vi "XNET Write (State Ethernet Sleep).vi"(0 "session in":refnum<k21>, 11 "error in (no error)":errorcluster) -> (4 "session out":refnum<k21>, 15 "error out":errorcluster)   [LabVIEW 2018]
doc: "Writes a request for the local Ethernet interface and its remote link partner to sleep. You can use this XNET Write VI with any input or output session for Ethernet."
uses:
  nixlvapi.dll
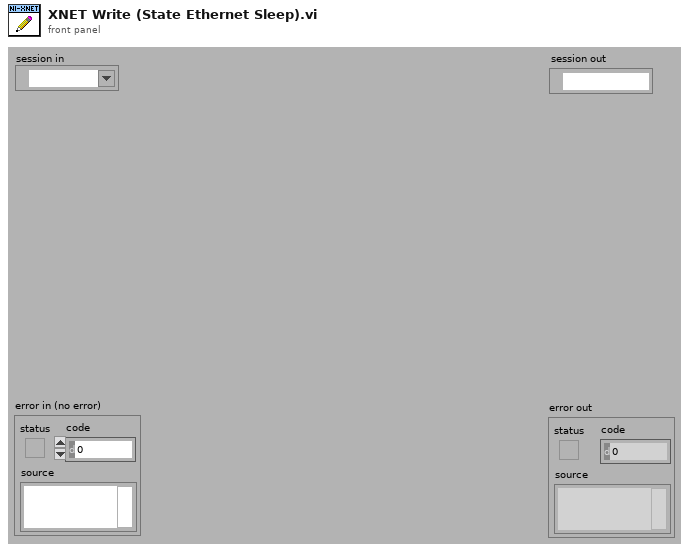
[diagram p1: front panel]
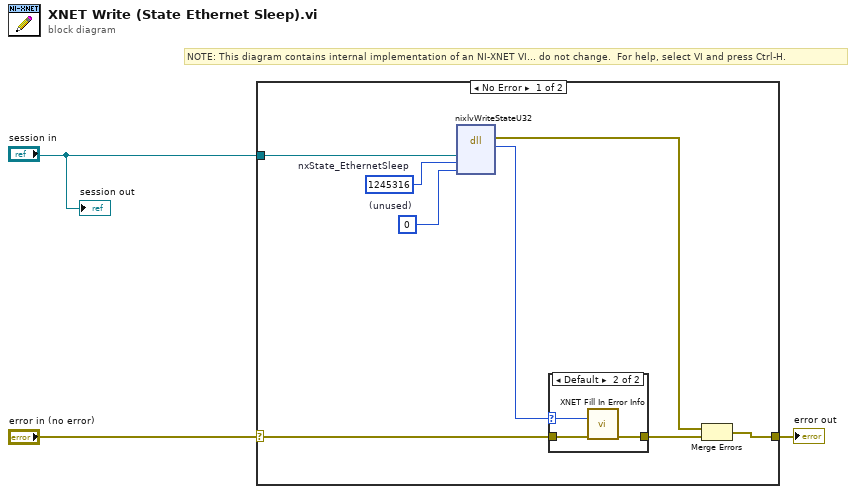
[diagram p0: block diagram]
diagram:
  # "NOTE: This diagram contains internal implementation of an NI-XNET VI... do not change.  For help, select VI and press Ctrl-H."
  n1 = case shown="No Error" "error in (no error)" {
    selector: "error in (no error)" -> [w10 w16]
    tunnel: "session in" -> [w11 _]
    tunnel: [w6 w16] -> w3
    frame No Error {
      w7 = u32 1245316  # nxState_EthernetSleep
      w8 = u32 0  # (unused)
      n2 = dll-call lib="nixlvapi.*" fn="nixlvWriteStateU32"("SessionRef"=w11, "StateID"=w7, "StateValue"=w8) -> (error out=w5:errorcluster, "return type"=w9:i32)  [unwired: 5 in, 2 out]
      n3 = case shown="Default" w9 {
        selector: w9 -> [_ w13]
        tunnel: w10 -> [w12 w14]
        tunnel: [w12 w15] -> w4
        frame 0 {
        }
        frame Default {
          n4 = call "XNET Fill In Error Info.vi"("status code"=w13, "error in"=w14) -> ("error out"=w15:errorcluster)  [unwired: 13 out]
        }
      }
      n5 = Merge Errors(w5, w4) -> (w6:errorcluster)
    }
    frame Error {
    }
  }
  "error out" <- w3
  "session out" <- "session in"
